vi "getDisplacement.vi"(8 "Freq_Cutoff":dbl, 9 "Samples to Average":i32, 10 "Samples":i32, 11 "Sampling Frequency":dbl) -> (2 "Frequency":dbl, 3 "max value":dbl)   [LabVIEW 2018]
panel:
  out "Iteration":i32
  out "XY Graph":cluster{"Y":dbl[], "Y":dbl[]}[](graph)
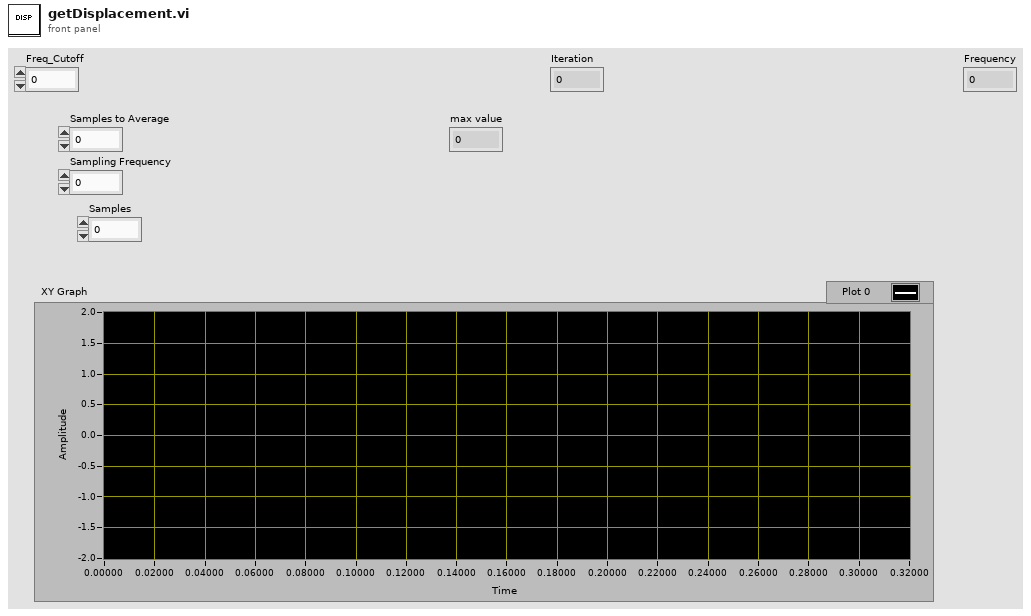
[diagram p1: front panel]
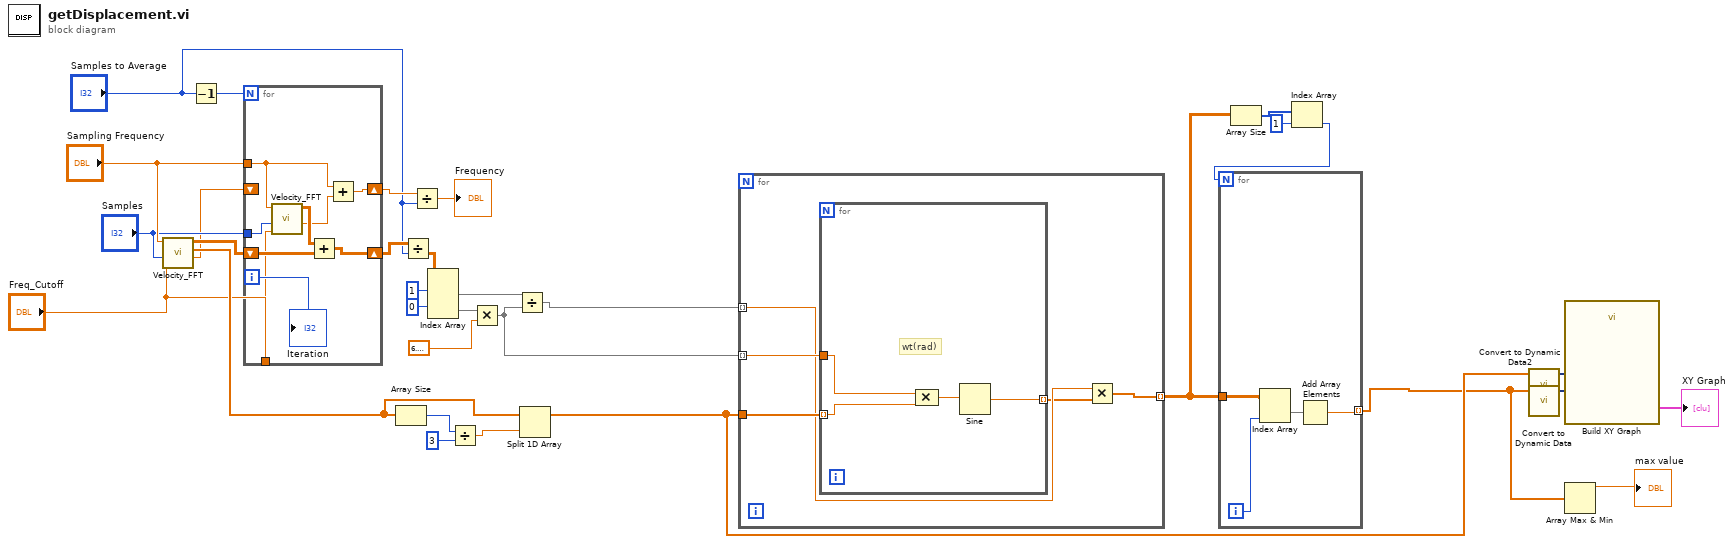
[diagram p0: block diagram]
diagram:
  n1 = call "Velocity_FFT.vi"("Freq_Cutoff"="Freq_Cutoff", "Samples"="Samples", "Sampling Frequency"="Sampling Frequency") -> ("Frequency"=w6:dbl, "t_vect"=w13:dbl[], "Peaks"=w24:dbl[][])  [unwired: 1 in, 3 out]
  n2 = Decrement(x="Samples to Average") -> (x-1=w28:i32)
  n3 = for {
    N: w28 -> [_]
    tunnel: "Sampling Frequency" -> [w34]
    shift-right: [w40] -> w29
    shift-left: w24 -> [w41]
    tunnel: "Samples" -> [w39]
    tunnel: "Freq_Cutoff" -> [w36]
    shift-right: [w35] -> w5
    shift-left: w6 -> [_]
    i -> [w37]
    n4 = call "Velocity_FFT.vi"("Freq_Cutoff"=w36, "Samples"=w39, "Sampling Frequency"=w34) -> ("Frequency"=w33:dbl, "Peaks"=w38:dbl[][])  [unwired: 1 in, 4 out]
    n5 = Add(x=w38, y=w41) -> (x+y=w40:dbl[][])
    n6 = Add(x=w34, y=w33) -> (x+y=w35:dbl)
    "Iteration" <- w37
  }
  n7 = Array Size(array=w13) -> (size(s)=w12:i32)
  n8 = Divide(x=w29, y="Samples to Average") -> (x/y=w30:dbl[][])
  n9 = Divide(x=w5, y="Samples to Average") -> (x/y=→"Frequency":dbl)
  n10 = Index Array(array=w30, index (row) #1=1 ("index (row)"), index (row) #2=0 ("index (row)")) -> (element #1=w25:dbl[], element #2=w23:dbl[])  [unwired: 2 in]
  n11 = Divide(x=w12, y=3) -> (x/y=w10:dbl)
  n12 = Multiply(x=w23, y=6.283185307179586) -> (x*y=w9:dbl[])
  n13 = Divide(x=w25, y=w9) -> (x/y=w2:dbl[])
  n14 = Split 1D Array(array=w13, index=w10) -> (first subarray=w14:dbl[])  [unwired: 1 out]
  n15 = for {
    tunnel: w9 -> [w45] mode=indexing
    tunnel: w2 -> [w44] mode=indexing
    tunnel: w14 -> [w46]
    tunnel: [w43] -> w19 mode=indexing
    n16 = for {
      tunnel: w46 -> [w50] mode=indexing
      tunnel: w45 -> [w49]
      tunnel: [w47] -> w42 mode=indexing
      # "wt(rad)"
      n17 = Compound Arithmetic op=MULTIPLY(w49, w50) -> (w48:dbl)
      n18 = Sine(x=w48) -> (sin(x)=w47:dbl)
    }
    n19 = Multiply(x=w44, y=w42) -> (x*y=w43:dbl[])
  }
  n20 = Array Size(array=w19) -> (size(s)=w18:i32[])
  n21 = Index Array(array=w18, index=1) -> (element=w16:i32)
  n22 = for {
    N: w16 -> [_]
    tunnel: w19 -> [w54]
    tunnel: [w51] -> w1 mode=indexing
    i -> [w53]
    n23 = Index Array(array=w54, index (col)=w53) -> (element=w52:dbl[])  [unwired: 1 in]
    n24 = Add Array Elements(numeric array=w52) -> (sum=w51:dbl)
  }
  n25 = call "Convert to Dynamic Data2"("Array"=w14) -> ("Dynamic Data Type"=w20:dynamicdata)  [unwired: 3 in]
  n26 = call "Convert to Dynamic Data"("Array"=w1) -> ("Dynamic Data Type"=w21:dynamicdata)  [unwired: 3 in]
  n27 = call "Build XY Graph"("Y Input"=w21, "X Input"=w20) -> ("XY Graph"=→"XY Graph":cluster{"X":dbl[], "Y":dbl[]}[])  [unwired: 8 in, 1 out]
  n28 = Array Max & Min(array=w1) -> (max value=→"max value":dbl)  [unwired: 3 out]
